vi "domeADB_monitorCommand_Echo.vi"(8 "error in (no error)":errorcluster, 11 "command_Echo_Ctl":T1) -> (0 "error out":errorcluster, 2 "function return":i32, 3 "command_Echo_Ctl out":T1)   [LabVIEW 2016, in "SALLV_domeADB.lvlib"]
doc: "int domeADB_shm_monitorCommand_EchoLV(domeADB_command_EchoLV *command_Echo_Ctl );"
uses:
  SALLV_domeADB.lvlib
  DataTypes/command_Echo.ctl
  SALLV_domeADB.so
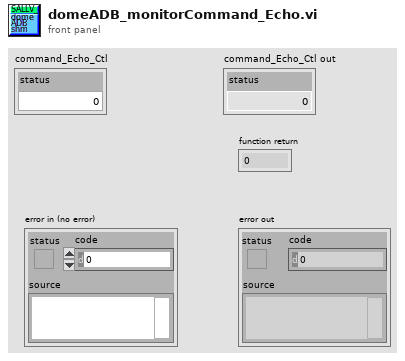
[diagram p1: front panel]
types:
  T1 = typedef "SALLV_domeADB.lvlib/command_Echo.ctl" = cluster{"status":i32}
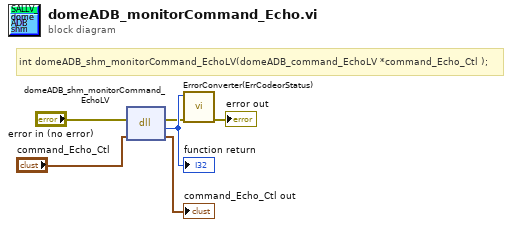
[diagram p0: block diagram]
diagram:
  # "int domeADB_shm_monitorCommand_EchoLV(domeADB_command_EchoLV *command_Echo_Ctl );"
  n1 = dll-call lib="home/andres/Desktop/SALLV_domeADB/SALLV_domeADB.*" fn="domeADB_shm_monitorCommand_EchoLV"(error in="error in (no error)", "command_Echo_Ctl"="command_Echo_Ctl") -> (error out=w2:errorcluster, w6:i32, "command_Echo_Ctl"=→"command_Echo_Ctl out":T1)  [unwired: 2 in, 1 out]
  "function return" <- w6
  n2 = call "ErrorConverter(ErrCodeorStatus).vi"("error in (no error)"=w2, "error code"=w6) -> ("error out"=→"error out":errorcluster)  [unwired: 9 in]
